vi "GetPeaksInRange.vi"(0 "Connection Cluster in":T1, 9 "Start Position":dbl, 11 "Fine range":dbl) -> (4 "Connection Cluster out":T1, 6 "Peak detected? right":bool, 8 "Peak (right)":dbl, 10 "Peak detected? left":bool, 15 "Peak (left)":dbl)   [LabVIEW 2013]
uses:
  Global.vi
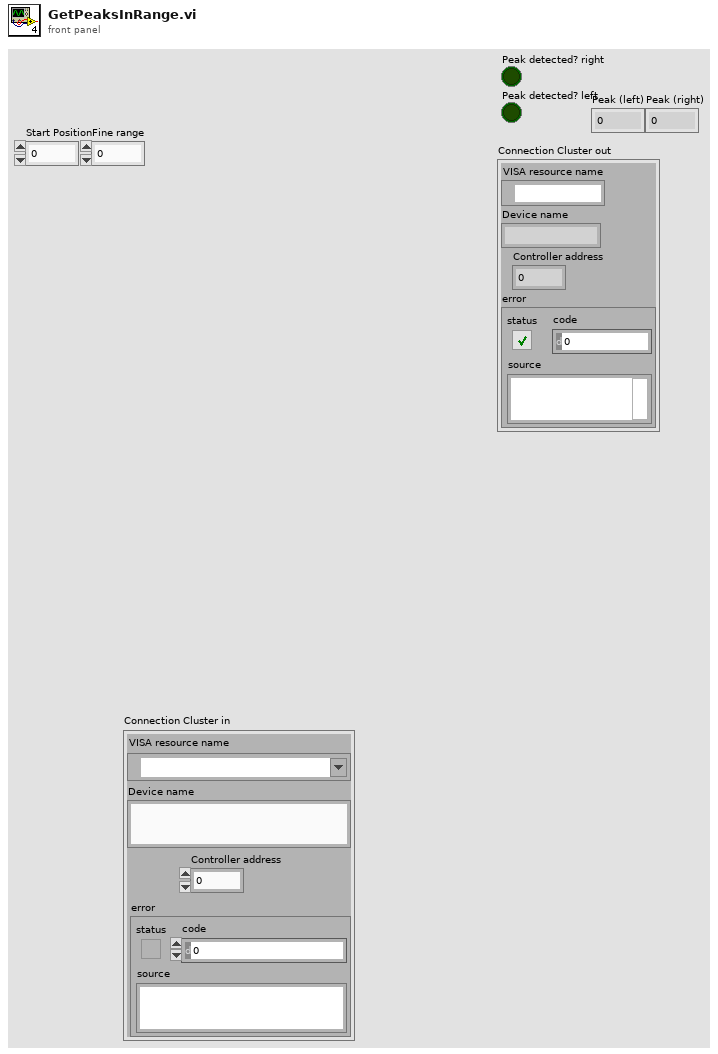
[diagram p1: front panel]
types:
  T1 = cluster{"VISA resource name":refnum<visa-resource-name>, "Device name":string, "Controller address":i32, "error":errorcluster}
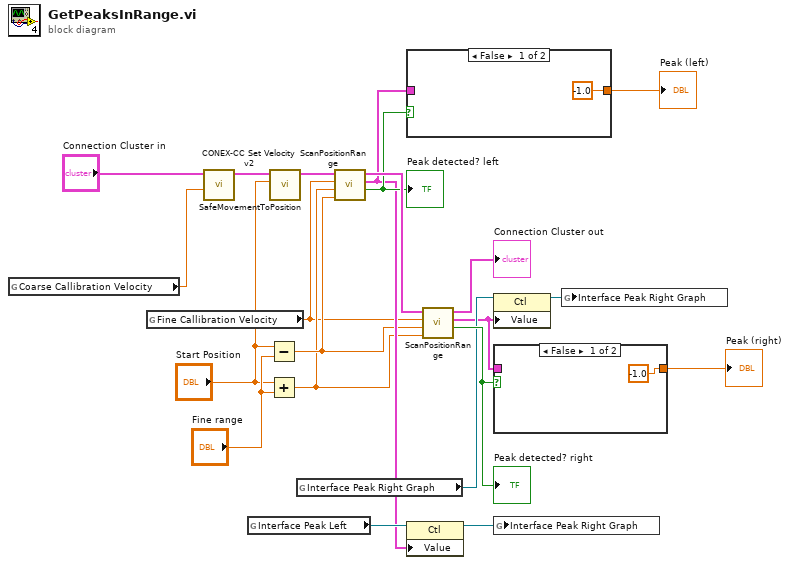
[diagram p0: block diagram]
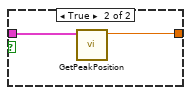
[diagram p2: hidden frame]
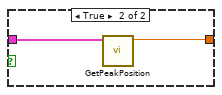
[diagram p3: hidden frame]
diagram:
  n1 = global read "Global.vi" "Coarse Callibration Velocity"() -> (w2:dbl)
  n2 = global read "Global.vi" "Fine Callibration Velocity"() -> (w1:dbl)
  n3 = call <userlib>:"CONEX-CC Set Velocity v2.vi"("Velocity"=w2, "Connection Cluster in"="Connection Cluster in") -> ("Connection Cluster out"=w6:T1)  [unwired: 9 in]
  n4 = global read "Global.vi" "Interface Peak Left"() -> (w11:refnum<vi>)
  n5 = Subtract(x="Start Position", y="Fine range") -> (x-y=w8:dbl)
  n6 = Add(x="Start Position", y="Fine range") -> (x+y=w7:dbl)
  n7 = call "SafeMovementToPosition.vi"("Target position"="Start Position", "Connection Cluster in"=w6) -> ("Connection Cluster out"=w4:T1)  [unwired: 9 in]
  n8 = global read "Global.vi" "Interface Peak Right Graph"() -> (w14:refnum<vi>)
  n9 = call "ScanPositionRange.vi"("Target position"=w8, "Start position"=w7, "Velocity"=w1, "Connection Cluster in"=w4) -> ("Peak detected?"=w17:bool, "output cluster"=w9:cluster{dbl[], dbl[]}, "Connection Cluster out"=w19:T1)  [unwired: 5 in]
  "Peak detected? left" <- w17
  n10 = case shown="False" w17 {
    tunnel: w9 -> [_ w24]
    tunnel: [-1.0 ("Peak position [mm]") w23] -> w18
    frame False {
    }
    frame True {
      n11 = call "GetPeakPosition.vi"("Input cluster"=w24) -> ("Peak position [mm]"=w23:dbl)  [unwired: 10 in]
    }
  }
  "Peak (left)" <- w18
  n12 = property class="Ctl"(reference=w11, "Value"=w9) -> (reference out=w10:refnum<vi>)  [unwired: 1 in, 1 out]
  n13 = call "ScanPositionRange.vi"("Target position"=w7, "Start position"=w8, "Velocity"=w1, "Connection Cluster in"=w19) -> ("Peak detected?"=w16:bool, "output cluster"=w12:cluster{dbl[], dbl[]}, "Connection Cluster out"=→"Connection Cluster out":T1)  [unwired: 5 in]
  "Peak detected? right" <- w16
  n14 = property class="Ctl"(reference=w14, "Value"=w12) -> (reference out=w13:refnum<vi>)  [unwired: 1 in, 1 out]
  n15 = case shown="False" w16 {
    tunnel: w12 -> [_ w27]
    tunnel: [-1.0 ("Peak position [mm]") w26] -> w15
    frame False {
    }
    frame True {
      n16 = call "GetPeakPosition.vi"("Input cluster"=w27) -> ("Peak position [mm]"=w26:dbl)  [unwired: 10 in]
    }
  }
  "Peak (right)" <- w15
  n17 = global write "Global.vi" "Interface Peak Right Graph"(w10) -> ()
  n18 = global write "Global.vi" "Interface Peak Right Graph"(w13) -> ()
